vi "Graphics-Draw Triangle (Picture).vi"(0 "picture in":picture, 7 "rect":T1, 11 "fill?(F)":bool, 12 "color(black)":u32(colorbox)=16711680, 13 "pen":T2) -> (4 "picture out":picture)   [LabVIEW 2020]
uses:
  <vilib>/Utility/miscctls.llb/LVRectTypeDef.ctl
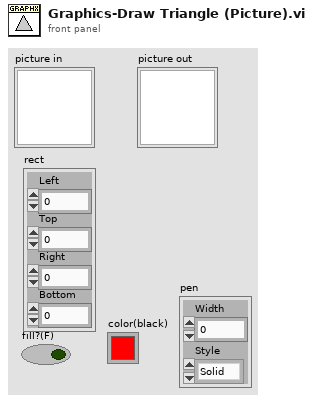
[diagram p1: front panel]
types:
  T1 = typedef "LVRectTypeDef.ctl" = cluster{"Left":i16, "Top":i16, "Right":i16, "Bottom":i16}
  T2 = cluster{"Width":u16, "Style":enum32{"Solid", "Dash", "Dot", "DashDot", "DashDotDot"}}
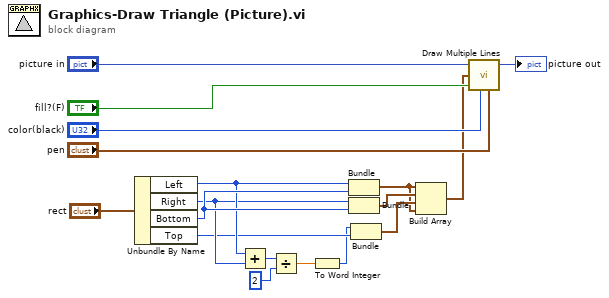
[diagram p0: block diagram]
diagram:
  n1 = Unbundle By Name("rect") -> ("Left"=w11:i16, "Right"=w10:i16, "Bottom"=w12:i16, "Top"=w7:i16)
  n2 = Add(x=w11, y=w10) -> (x+y=w9:i16)
  n3 = Divide(x=w9, y=2) -> (x/y=w6:dbl)
  n4 = To Word Integer(number=w6) -> (16bit integer=w5:i16)
  n5 = Bundle("Left"=w11, "Bottom"=w12) -> (w1:cluster{"Left":i16, "Bottom":i16})  [unwired: 1 in]
  n6 = Bundle("Right"=w10, "Bottom"=w12) -> (w4:cluster{"Right":i16, "Bottom":i16})  [unwired: 1 in]
  n7 = Bundle(w5, "Top"=w7) -> (w3:cluster{i16, "Top":i16})  [unwired: 1 in]
  n8 = Build Array(w1, w4, w3, w1) -> (w2:cluster{"Left":i16, "Bottom":i16}[])
  n9 = call <vilib>:"Draw Multiple Lines.vi"("picture"="picture in", "line endpoints"=w2, "fill?(F)"="fill?(F)", "color(black)"="color(black)", "pen"="pen") -> ("new picture"=→"picture out":picture)  [unwired: 4 in]
